vi "Acquire-a.vi"() -> (4 "Waveform Chart":dbl(graph))   [LabVIEW 2020]
uses:
  SubVI/Stop Global Variable.vi
  SubVI/Numeric Global variable.vi
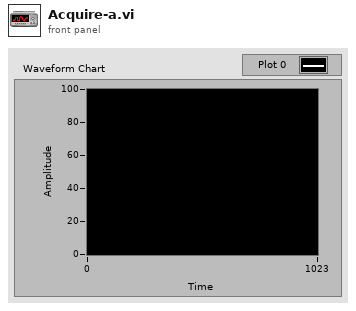
[diagram p1: front panel]
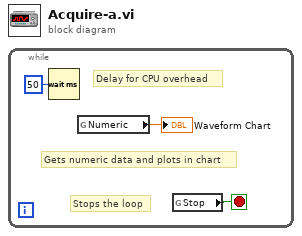
[diagram p0: block diagram]
diagram:
  n1 = while {
    stop <- w1 stop-if-true
    # "Delay for CPU overhead"
    # "Stops the loop"
    # "Gets numeric data and plots in chart"
    n2 = Wait (ms)(milliseconds to wait=u32 50) -> ()  [unwired: 1 out]
    n3 = global read "Numeric Global variable.vi" "Numeric"() -> (→"Waveform Chart":dbl)
    n4 = global read "Stop Global Variable.vi" "Stop"() -> (w1:bool)
  }
